vi "Close2000.vi"   [LabVIEW 2013]
uses:
  <vilib>/Heliosphere Research LLC/Advanced Plotting Toolkit/Advanced Plotting Toolkit.lvlib
types:
  T1 = typedef "Advanced Plotting Toolkit.lvlib/PlotID.ctl" = i32
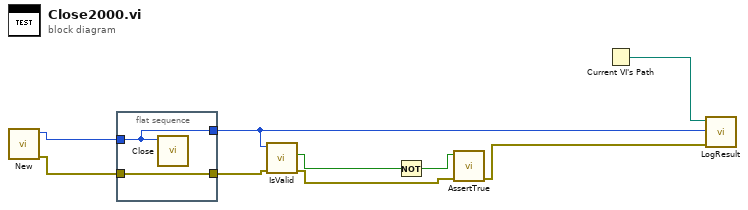
[diagram p0: block diagram]
diagram:
  n1 = call <vilib>:"New.vi"() -> ("error out"=w7:errorcluster, "Plot ID"=w8:T1)  [unwired: 10 in]
  n2 = flat-sequence {
    tunnel: w8 -> [w10]
    tunnel: w7 -> [w11]
    tunnel: [w11] -> w6
    tunnel: [w10] -> w1
    frame #0 {
      n3 = call <vilib>:"Close.vi"("Plot ID"=w10) -> ()  [unwired: 11 in]
    }
  }
  n4 = call <vilib>:"IsValid.vi"("error in (no error)"=w6, "Plot ID"=w1) -> ("error out"=w3:errorcluster, "Valid?"=w5:bool)  [unwired: 7 in, 1 out]
  n5 = Not(x=w5) -> (.not. x?=w4:bool)
  n6 = call "AssertTrue.vi"("error in (no error)"=w3, "Value"=w4) -> ("error out"=w2:errorcluster)  [unwired: 9 in]
  n7 = Current VI's Path() -> (path=w9:path)
  n8 = call "LogResult.vi"("Test Result"=w2, "Test Artifact"=w1, "VI Path"=w9) -> ()  [unwired: 9 in]
